vi "ddr_write.vi"(5 "COM":bool, 7 "VISA name":refnum<visa-resource-name>, 9 "pbydata":u8[](array[numeric]), 10 "dwLen":u32, 11 "dwStartAddr":u32) -> (3 "return":i32)   [LabVIEW 2016]
panel:
  in  "tVdCmdHeader":T1
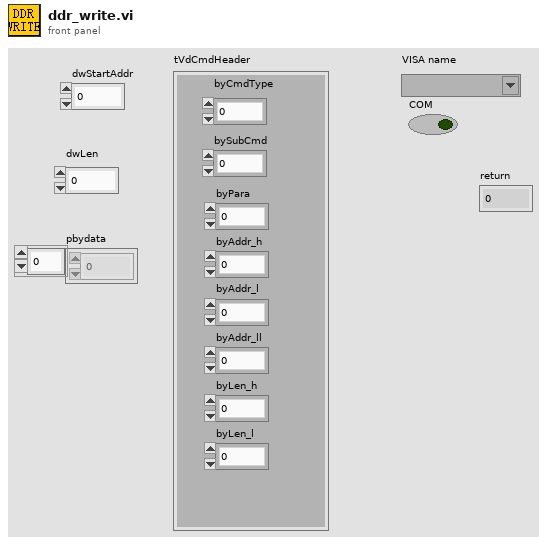
[diagram p1: front panel]
types:
  T1 = cluster{"byCmdType":u8, "bySubCmd":u8, "byPara":u8, "byAddr_h":u8, "byAddr_l":u8, "byAddr_ll":u8, "byLen_h ":u8, "byLen_l":u8}
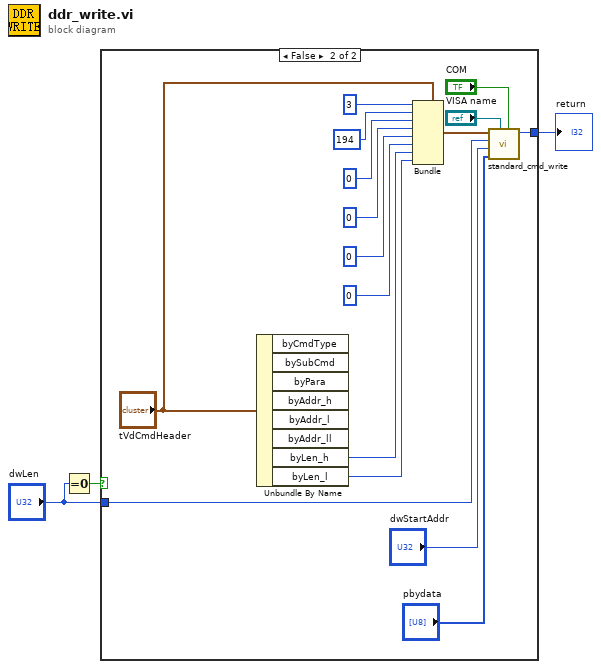
[diagram p0: block diagram]
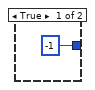
[diagram p2: hidden frame]
diagram:
  n1 = Equal To 0?(x="dwLen") -> (x = 0?=w2:bool)
  n2 = case shown="False" w2 {
    tunnel: [-1 w8] -> w3
    tunnel: "dwLen" -> [_ w7]
    frame True {
    }
    frame False {
      n3 = Unbundle By Name("tVdCmdHeader") -> ("byLen_h"=w17:u8, "byLen_l"=w16:u8)  [unwired: 6 out]
      n4 = Bundle(cluster="tVdCmdHeader", "byCmdType"=u8 3, "bySubCmd"=u8 194, "byPara"=u8 0, "byAddr_h"=u8 0, "byAddr_l"=u8 0, "byAddr_ll"=u8 0, "byLen_h"=w17, "byLen_l"=w16) -> (w15:T1)
      n5 = call "standard_cmd_write.vi"("COM"="COM", "VISA name"="VISA name", "data"="pbydata", "dwLen"="dwStartAddr", "dwAddr"=w7, "cmd_std_header_t"=w15) -> ("return"=w8:i32)  [unwired: 5 in]
    }
  }
  "return" <- w3
